vi "Insert Value (Value).vi"(7 "key":string, 8 "error in (no error)":errorcluster, 10 "JSON Value in":refnum<class "JSON Value.lvclass">, 11 "JSON Value in":refnum<class "JSON Value.lvclass">) -> (0 "error out":errorcluster, 1 "replaced":bool, 3 "JSON Value out":refnum<class "JSON Value.lvclass">)   [LabVIEW 2016, in "JSON Value.lvclass"]
uses:
  JSON Value.lvclass
  JSON Value.lvclass/JSON Value.ctl
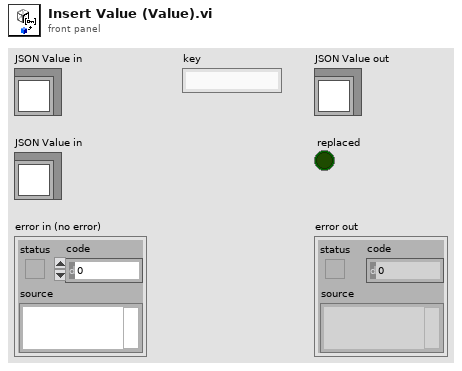
[diagram p1: front panel]
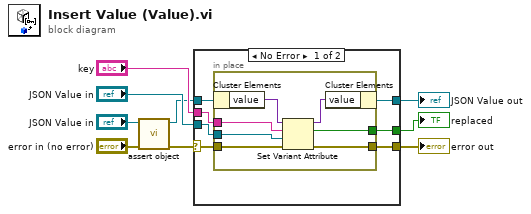
[diagram p0: block diagram]
diagram:
  n1 = call "assert object.vi"("error in (no error)"="error in (no error)", "JSON Value in"="JSON Value in") -> ("error out"=w3:errorcluster, "JSON Value out"=w1:refnum<class "JSON Value.lvclass">)  [unwired: 8 in]
  n2 = case shown="No Error" w3 {
    selector: w3 -> [w10 w25]
    tunnel: [w13 w25] -> w5
    tunnel: [w16 w24] -> w7
    tunnel: w1 -> [w11 w24]
    tunnel: "key" -> [w15 _]
    tunnel: "JSON Value in" -> [w14 _]
    tunnel: [w12 _] -> w6
    frame No Error {
      n3 = in-place {
        in-place-border: w15 -> [w22]
        in-place-border: w14 -> [w18]
        in-place-border: w10 -> [w19]
        in-place-border: [w20] -> w13
        in-place-border: [w17] -> w12
        n4 = in-place-cluster #1(w11) -> ("value"=w23:variant)
        n5 = Set Variant Attribute(Variant=w23, name=w22, value=w18, error in=w19) -> (Variant out=w21:variant, replaced=w17:bool, error out=w20:errorcluster)
        n6 = in-place-cluster #1("value"=w21) -> (w16:refnum<class "JSON Value.lvclass">)
      }
    }
    frame Error {
    }
  }
  "error out" <- w5
  "JSON Value out" <- w7
  "replaced" <- w6
